vi "validate line configuration.vi"(7 "module":refnum<class "OPC UA Client configuration.lvclass">, 11 "Mappings in":T1 {"Line"."OPC UA Data Type" items=["Boolean"=1, "SByte"=2, "Byte"=3, "Int16"=4, "UInt16"=5, "Int32"=6, "UInt32"=7, "Int64"=8, "UInt64"=9, "Float"=10, "Double"=11, "String"=12, "DateTime"=13, "ByteString"=15, "Array of Boolean"=101, "Array of SByte"=102, "Array of Byte"=103, "Array of Int16"=104, "Array of UInt16"=105, "Array of Int32"=106, "Array of UInt32"=107, "Array of Int64"=108, "Array of UInt64"=109, "Array of Float"=110, "Array of Double"=111, "Array of String"=112, "Array of DateTime"=113, "Array of ByteString"=115]}) -> (1 "valid?":bool, 2 "errors":string, 3 "Mappings out":T1 {"Line"."OPC UA Data Type" items=["Boolean"=1, "SByte"=2, "Byte"=3, "Int16"=4, "UInt16"=5, "Int32"=6, "UInt32"=7, "Int64"=8, "UInt64"=9, "Float"=10, "Double"=11, "String"=12, "DateTime"=13, "ByteString"=15, "Array of Boolean"=101, "Array of SByte"=102, "Array of Byte"=103, "Array of Int16"=104, "Array of UInt16"=105, "Array of Int32"=106, "Array of UInt32"=107, "Array of Int64"=108, "Array of UInt64"=109, "Array of Float"=110, "Array of Double"=111, "Array of String"=112, "Array of DateTime"=113, "Array of ByteString"=115]})   [LabVIEW 2013, in "OPC UA Client editor node.lvclass"]
uses:
  OPC UA Client editor node.lvclass
  Mappings.ctl
  <vilib>/NI/Tag Bus Module Framework/channel/TBM channel.lvclass
  module/configuration/Line.ctl
  module/configuration/OPC UA Data Type.ctl
  Map.ctl
  module/configuration/OPC UA Client configuration.lvclass
  <vilib>/NI/Tag Bus/tag/tag descriptor.lvclass/tag descriptor.ctl
  <vilib>/NI/Tag Bus/tag/read tag name.vi
  <vilib>/NI/Tag Bus/tag/read data type.vi
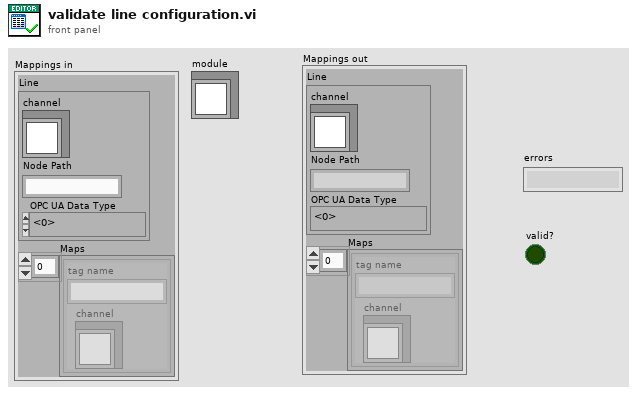
[diagram p1: front panel]
types:
  T1 = typedef "OPC UA Client editor node.lvclass/Mappings.ctl" = cluster{"Line":T2, "Maps":T4[]}
  T2 = typedef "OPC UA Client configuration.lvclass/Line.ctl" = cluster{"channel":refnum<class "TBM channel.lvclass">, "Node Path":string, "OPC UA Data Type":T3}
  T3 = typedef "OPC UA Client configuration.lvclass/OPC UA Data Type.ctl" = u16
  T4 = typedef "OPC UA Client editor node.lvclass/Map.ctl" = cluster{"channel":refnum<class "TBM channel.lvclass">, "tag name":string}
  T5 = typedef "tag bus.lvlib/tag descriptor.lvclass/Data Type.ctl" = enum16{"Double", "Single", "I64", "I32", "I16", "I8", "U64", "U32", "U16", "U8", "Boolean", "String", "Array of Double", "Array of Single", "Array of I64", "Array of I32", "Array of I16", "Array of I8", "Array of U64", "Array of U32", "Array of U16", "Array of U8", "Array of Boolean", "Array of String"}
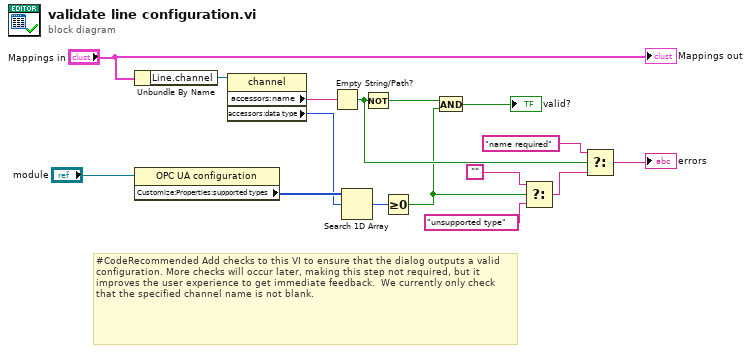
[diagram p0: block diagram]
diagram:
  # "#CodeRecommended Add checks to this VI to ensure that the dialog outputs a valid configuration. More checks will occur later, making this step not required, but it improves the user experience to get immediate feedback.  We currently only check that the specified channel name is not blank."
  n1 = Unbundle By Name("Mappings in") -> ("Line.channel"=w15:refnum<class "TBM channel.lvclass">)
  n2 = property class="OPC UA configuration"(reference="module") -> ("Customize:Properties:supported types"=w11:T5[])  [unwired: 1 in, 2 out]
  n3 = property class="channel"(reference=w15) -> ("accessors:name"=w14:string, "accessors:data type"=w10:T5)  [unwired: 1 in, 2 out]
  n4 = Empty String/Path?(string/path=w14) -> (empty?=w7:bool)
  n5 = Search 1D Array(1D array=w11, element=w10) -> (index of element=w8:i32)  [unwired: 1 in]
  n6 = Not(x=w7) -> (.not. x?=w13:bool)
  n7 = Greater Or Equal To 0?(x=w8) -> (x >= 0?=w4:bool)
  n8 = And(x=w13, y=w4) -> (x .and. y?=→"valid?":bool)
  n9 = Select(t="", s=w4, f="unsupported type") -> (s? t:f=w2:string)
  n10 = Select(t="name required", s=w7, f=w2) -> (s? t:f=→"errors":string)
  "Mappings out" <- "Mappings in"
